vi "Eagle_RT Scanner Timing Tests 1.vi"() -> ()   [LabVIEW 2015]
uses:
  <vilib>/Platform/TimedLoop/XDataNode/timing_clust.ctl
  <vilib>/Platform/TimedLoop/XDataNode/nitl_modes.ctl
  <vilib>/Platform/TimedLoop/XDataNode/wakeup.ctl
  <vilib>/FPGAPlugInAG/cRIO-9030/niLvFpga_Open_cRIO-9030.vi
  <vilib>/rvi/interface/common/dynamic/niFpgaDynamicAddResources.vi
  <vilib>/FPGAPlugInAG/Dynamic/niLvFpga_Run_Dynamic.vi
  <vilib>/Utility/error.llb/Error Cluster From Error Code.vi
  <vilib>/rvi/errors/niLvFpgaAdjustHostInterfaceError.vi
  <vilib>/rvi/interface/nirviOpenFPGA/nirviOpenFPGA.xnode
  FPGA Bitfiles/BELKINEAGLEGUI_FPGATarget_EagleFPGAScanner_juOkZGXIgM0.lvbitx
  Eagle_FPGA Scanner Control.vi
  <vilib>/rvi/interface/nirviMethod/nirviMethod.xnode
  <vilib>/rvi/interface/nirviReadWriteControl/nirviReadWriteControl.xnode
  <vilib>/Platform/TimedLoop/XDataNode/XDataNode.xnode
  NiFpgaLv.dll
  <vilib>/rvi/interface/Simulation/niFpgaSimulationCallBeginRW.vi
  <vilib>/Platform/TimedLoop/XDataNode/XDNodeRunTimeDep.lvlib
panel:
  in  "file path (use dialog)":path=path "c:/AriehData/Data1.csv"
  out "error out":errorcluster
  in  "X=True":bool
  in  "Manual Target":fxp<+/-,20,5>
  out "XY Graph":cluster{dbl[], dbl[]}(graph)
  out "Array":fxp<+/-,20,5>[](array[numeric])
  in  "Manual Start":fxp<+/-,20,5>
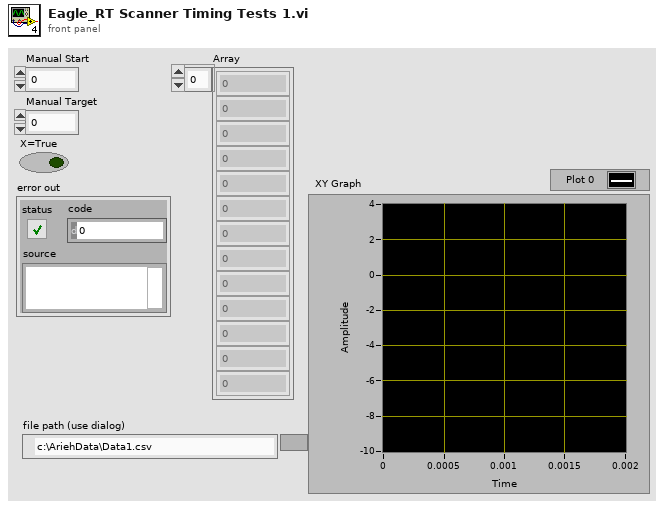
[diagram p1: front panel]
types:
  T1 = enum16{"open", "replace", "create", "open or create", "replace or create", "replace or create with confirmation"}
  T2 = typedef "XDNodeRunTimeDep.lvlib/timing_clust.ctl" = cluster{"Expected End [f-1]":u64, "Actual End [f-1]":u64, "Finished Late? [f-1]":bool, "Expected End [i-1]":u64, "Actual End [i-1]":u64, "Finished Late? [i-1]":bool, "Expected Start [i]":u64, "Actual Start [i]":u64, "Expected Start [f]":u64, "Actual Start [f]":u64, "Source Name":string, "Structure Name":string, "Period":i64, "Deadline":i64, "Offset":i64, "Start":i64, "Priority":i32, "Timeout":i32, "Mode":T3, "Wakeup Reason":T4, "Error":errorcluster, "Source Type":string, "Secondary Source Type":string, "Global End Time":u64, "Global Start Time":u64, "Frame Duration":u64, "Iteration Duration":u64, "Assigned CPU":i32, "I/O Scan Engine Mode":u32}
  T3 = typedef "XDNodeRunTimeDep.lvlib/nitl_modes.ctl" = enum32{"No Change", "Process missed periods, maintain original phase", "Discard missed periods, maintain original phase", "Process missed periods, ignore original phase", "Discard missed periods, ignore original phase"}
  T4 = typedef "XDNodeRunTimeDep.lvlib/wakeup.ctl" = enum32{"Normal", "Aborted", "Asynchronous wakeup", "Timing source error", "Timed loop error", "Timeout"}
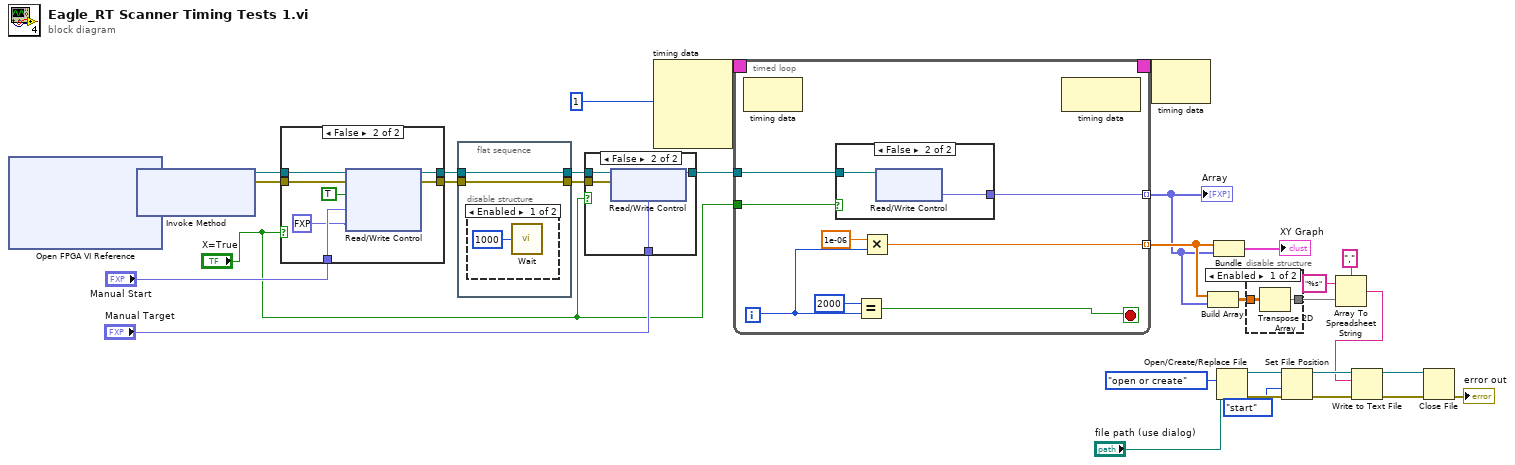
[diagram p0: block diagram]
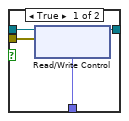
[diagram p3: hidden frame]
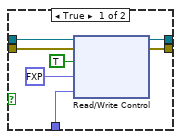
[diagram p4: hidden frame]
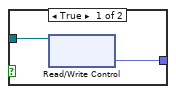
[diagram p5: hidden frame]
diagram:
  n1 = xnode "Open FPGA VI Reference"() -> ("FPGA VI Reference Out"=w33:refnum<k20>, "error out"=w30:errorcluster)  [unwired: 2 in]
  n2 = xnode "Invoke Method"("FPGA VI Reference In"=w33, "error in"=w30) -> ("FPGA VI Reference Out"=w32:refnum<k20>, "error out"=w31:errorcluster)  [unwired: 1 in]
  n3 = case shown="False" "X=True" {
    tunnel: w32 -> [w40 w47]
    tunnel: w31 -> [w39 w46]
    tunnel: [w36 w44] -> w29
    tunnel: "Manual Start" -> [w35 w42]
    tunnel: [w34 w43] -> w27
    frame True {
      n4 = xnode "Read/Write Control"("FPGA VI Reference In"=w40, "error in"=w39, "Manual"=TRUE, "Manual VY"=fxp<+/-,20,5> 0.0, "Manual VX"=w35) -> ("FPGA VI Reference Out"=w34:refnum<k20>, "error out"=w36:errorcluster)
    }
    frame False {
      n5 = xnode "Read/Write Control"("FPGA VI Reference In"=w47, "error in"=w46, "Manual"=TRUE, "Manual VY"=w42, "Manual VX"=fxp<+/-,20,5> 0.0 ("Manual VY")) -> ("FPGA VI Reference Out"=w43:refnum<k20>, "error out"=w44:errorcluster)
    }
  }
  n6 = flat-sequence {
    tunnel: [w49] -> w21
    tunnel: w29 -> [w49]
    tunnel: [w48] -> w22
    tunnel: w27 -> [w48]
    frame #0 {
      n7 = disable-structure shown="Enabled" {
        frame Enabled {
          n8 = call "Wait"("Count(mSec)"=u32 1000) -> ()  [unwired: 1 out]
        }
        frame Disabled {
        }
      }
    }
  }
  n9 = case shown="False" "X=True" {
    tunnel: w22 -> [w54 w58]
    tunnel: w21 -> [w53 w57]
    tunnel: [w52 w56] -> w20
    tunnel: "Manual Target" -> [w51 w55]
    frame True {
      n10 = xnode "Read/Write Control"("FPGA VI Reference In"=w54, "error in"=w53, "Manual VX"=w51) -> ("FPGA VI Reference Out"=w52:refnum<k20>)  [unwired: 1 out]
    }
    frame False {
      n11 = xnode "Read/Write Control"("FPGA VI Reference In"=w58, "error in"=w57, "Manual VY"=w55) -> ("FPGA VI Reference Out"=w56:refnum<k20>)  [unwired: 1 out]
    }
  }
  n12 = node-c288(i64 1 ("Period")) -> (w26:T2)  [unwired: 3 in]
  n13 = timed-loop {
    timing: w26 -> [_]
    timing-out: [_] -> w25
    tunnel: w20 -> [w66]
    tunnel: [w65] -> w10 mode=indexing
    tunnel: [w60] -> w11 mode=indexing
    tunnel: "X=True" -> [w59]
    i -> [w62]
    stop <- w63 stop-if-true
    n14 = node-c288() -> ()  [unwired: 1 in, 1 out]
    n15 = case shown="False" w59 {
      tunnel: w66 -> [w68 w70]
      tunnel: [w67 w69] -> w65
      frame True {
        n16 = xnode "Read/Write Control"("FPGA VI Reference In"=w68) -> ("X READ 2"=w67:fxp<+/-,20,5>)  [unwired: 1 in, 2 out]
      }
      frame False {
        n17 = xnode "Read/Write Control"("FPGA VI Reference In"=w70) -> ("Y READ 2"=w69:fxp<+/-,20,5>)  [unwired: 1 in, 2 out]
      }
    }
    n18 = Equal?(x=2000, y=w62) -> (x = y?=w63:bool)
    n19 = Multiply(x=1e-06, y=w62) -> (x*y=w60:dbl)
    n20 = node-c288() -> ()  [unwired: 1 in, 1 out]
  }
  "Array" <- w10
  n21 = node-c288(w25) -> ()  [unwired: 1 out]
  n22 = Build Array(w11, w10) -> (w3:dbl[][])
  n23 = Bundle(w11, w10) -> (→"XY Graph":cluster{dbl[], fxp<+/-,20,5>[]})  [unwired: 1 in]
  n24 = Open/Create/Replace File(file path (use dialog)="file path (use dialog)", operation (0:open)=T1."open or create") -> (refnum out=w16:refnum<file>, error out=w15:errorcluster)  [unwired: 4 in, 1 out]
  n25 = disable-structure shown="Enabled" {
    disable-tunnel: w3 -> [w74 w75]
    disable-tunnel: [w73 w75] -> w2
    frame Enabled {
      n26 = Transpose 2D Array(2D array=w74) -> (transposed array=w73:dbl[][])
    }
    frame Disabled {
    }
  }
  n27 = Set File Position(refnum=w16, from (0:start)=enum16{"start", "end", "current"}."start", error in=w15) -> (refnum out=w12:refnum<file>, error out=w13:errorcluster)  [unwired: 1 in]
  n28 = Array To Spreadsheet String(delimiter (Tab)=",", array=w2, 3:"%s" ("format string")) -> (spreadsheet string=w1:string)
  n29 = Write to Text File(file (use dialog)=w12, text=w1, error in=w13) -> (refnum out=w6:refnum<file>, error out=w7:errorcluster)  [unwired: 1 in, 1 out]
  n30 = Close File(refnum=w6, error in=w7) -> (error out=→"error out":errorcluster)  [unwired: 1 out]
